vi "servo_test.vi"() -> ()   [LabVIEW 2019]
uses:
  WSCbot_V3_Toolkit.lvlibp/WSCBOTV3_Toolkit/IO/LowLevel/IO_Chanel_DIO.ctl
  WSCbot_V3_Toolkit.lvlibp/WSCBOTV3_Toolkit/IO/LowLevel/PWM.vi
  WSCbot_V3_Toolkit.lvlibp
panel:
  out "pwm":dbl
  in  "IO_Chanel":T1
  in  "angle":dbl(slide)=1287.564766839378 scale=500.0..2500.0
  in  "Stop Button":bool
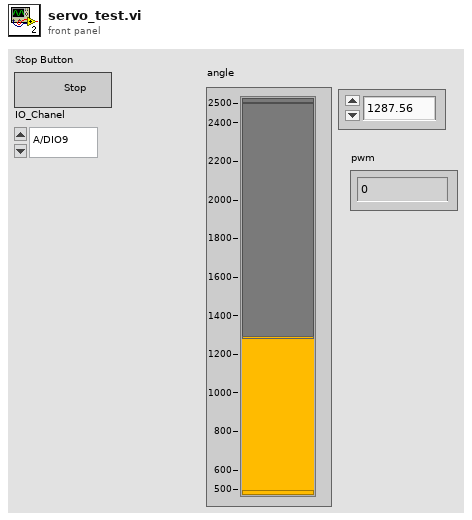
[diagram p1: front panel]
types:
  T1 = typedef "WSCbot_V3_Toolkit.lvlibp/IO_Chanel_DIO.ctl" = enum16{"A/DIO9", "A/DIO10", "C/DIO0", "C/DIO1", "C/DIO2", "C/DIO3", "C/DIO4", "C/DIO5", "C/DIO6"}
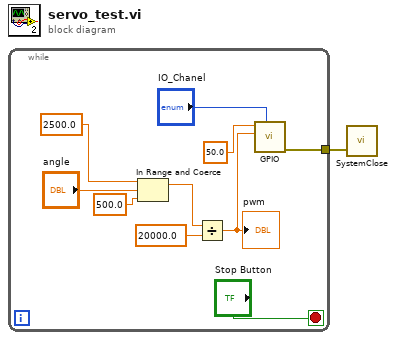
[diagram p0: block diagram]
diagram:
  n1 = while {
    tunnel: [w7] -> w1
    stop <- "Stop Button" stop-if-true
    n2 = In Range and Coerce(upper limit=2500.0, x="angle", lower limit=500.0) -> (coerced(x)=w4:dbl)  [unwired: 1 out]
    n3 = Divide(x=w4, y=20000.0) -> (x/y=w5:dbl)
    "pwm" <- w5
    n4 = call-poly "GPIO.vi"("IO_Chanel"="IO_Chanel", "DutyCycle"=w5, "Frequency(Hz)"=50.0) -> ("error out"=w7:errorcluster)  [unwired: 8 in]
  }
  n5 = call "SystemClose.vi"("error in"=w1) -> ()  [unwired: 2 in, 1 out]
